vi "Dual State Press Change.vi"(1 "Enable/Disable":bool) -> (0 "Enabled":bool)   [LabVIEW 2011]
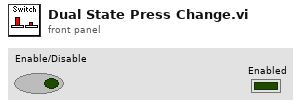
[diagram p1: front panel]
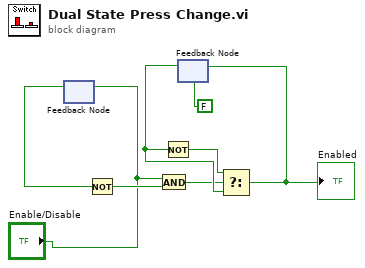
[diagram p0: block diagram]
diagram:
  n1 = feedback #1() -> (w2:bool)  [unwired: 1 in]
  n2 = feedback-in #1("Enable/Disable") -> ()
  n3 = Not(x=w2) -> (.not. x?=w3:bool)
  n4 = And(x="Enable/Disable", y=w3) -> (x .and. y?=w5:bool)
  n5 = feedback #2(FALSE) -> (w7:bool)
  n6 = Not(x=w7) -> (.not. x?=w6:bool)
  n7 = Select(t=w6, s=w5, f=w7) -> (s? t:f=w8:bool)
  "Enabled" <- w8
  n8 = feedback-in #2(w8) -> ()
